vi "Piece_Init.vi"(8 "error in (no error)":errorcluster, 10 "pieceColor":T1, 11 "object in":refnum<class "Piece.lvclass">) -> (0 "error out":errorcluster, 3 "object out":refnum<class "Piece.lvclass">)   [LabVIEW 2020, in "Piece.lvclass"]
doc: "Initializes the piece"
uses:
  Piece.lvclass
  typedefs/pieceColor.ctl
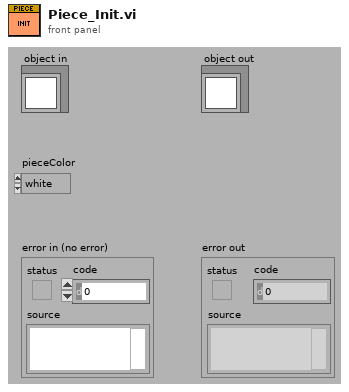
[diagram p1: front panel]
types:
  T1 = typedef "pieceColor.ctl" = enum16{"white", "black"}
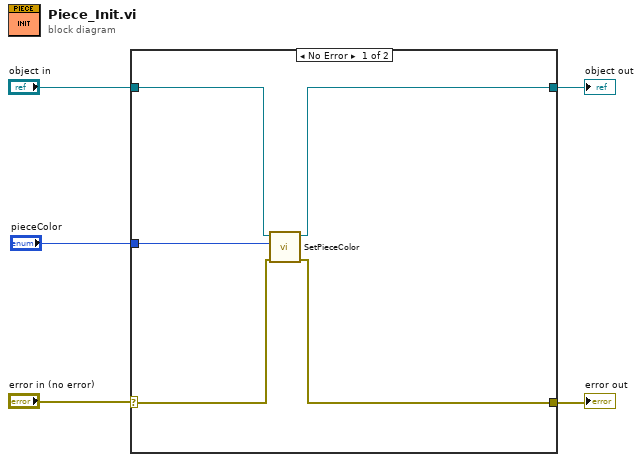
[diagram p0: block diagram]
diagram:
  n1 = case shown="No Error" "error in (no error)" {
    selector: "error in (no error)" -> [w7 w11]
    tunnel: "object in" -> [w10 w12]
    tunnel: [w9 w12] -> w4
    tunnel: [w6 w11] -> w2
    tunnel: "pieceColor" -> [w8 _]
    frame No Error {
      n2 = call-dynamic "SetPieceColor.vi"("error in (no error)"=w7, "pieceColor"=w8, "object in"=w10) -> ("error out"=w6:errorcluster, "object out"=w9:refnum<class "Piece.lvclass">)  [unwired: 7 in]
    }
    frame Error {
    }
  }
  "object out" <- w4
  "error out" <- w2
